vi "InTake Finish.vi"   [LabVIEW 2013]
types:
  T1 = typedef "WPI_MotorControlDeviceRef.ctl" = cluster{"DeviceStatus":errorcluster, "Type":enum16{"PWM", "CAN"}, "PWM":cluster{"Digital Module":T2, "PWM Channel":T3, "DeadBand":T4}, "CAN":cluster{"Device Number":u8, "Control Mode":T5, "Semaphore":T6, "Max Vout":dbl}, "Invert":bool, "TransformRef":T7, "InvTransformRef":T7}
  T2 = typedef "FPGA_TypedefDigitalModule.ctl" = enum16{"Digital Module 1", "Digital Module 2"}
  T3 = typedef "FPGA_DIOPWMChannel.ctl" = enum8{"PWM 1", "PWM 2", "PWM 3", "PWM 4", "PWM 5", "PWM 6", "PWM 7", "PWM 8", "PWM 9", "PWM 10", "Invalid"}
  T4 = typedef "WPI_PWMDeadband.ctl" = cluster{"Name":string, "maxPositivePwm":i32, "minPositivePwm":i32, "centerPwm":i32, "maxNegativePwm":i32, "minNegativePwm":i32, "angularRange":u16}
  T5 = typedef "WPI_CANJaguar_ControlMode.ctl" = enum8{"Percent VBus", "Current", "Speed", "Position", "Voltage"}
  T6 = typedef "Semaphore RefNum" = refnum<k1>
  T7 = typedef "WPI_PWMTransform_ConPane.ctl" = refnum<vi>
  T8 = typedef "WPI_DigitalInputDevRef.ctl" = cluster{"DevStatus":errorcluster, "DIO Channel":T9, "Digital Module":T2}
  T9 = typedef "FPGA_DIOChannel.ctl" = enum8{"DIO 1", "DIO 2", "DIO 3", "DIO 4", "DIO 5", "DIO 6", "DIO 7", "DIO 8", "DIO 9", "DIO 10", "DIO 11", "DIO 12", "DIO 13", "DIO 14", "Invalid"}
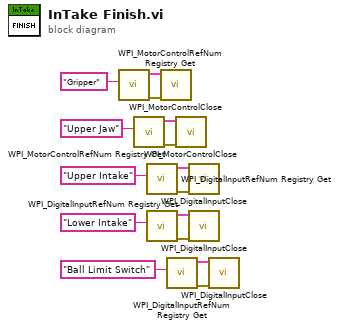
[diagram p0: block diagram]
diagram:
  n1 = call <vilib>:"WPI_MotorControlRefNum Registry Get.vi"("refnum name"="Gripper") -> ("error out"=w10:errorcluster, "MotorControlDevRef"=w9:T1)  [unwired: 9 in]
  n2 = call <vilib>:"WPI_MotorControlRefNum Registry Get.vi"("refnum name"="Upper Jaw") -> ("error out"=w8:errorcluster, "MotorControlDevRef"=w7:T1)  [unwired: 9 in]
  n3 = call <vilib>:"WPI_DigitalInputRefNum Registry Get.vi"("refnum name"="Upper Intake") -> ("error out"=w6:errorcluster, "DigitalInputDevRef"=w5:T8)  [unwired: 9 in]
  n4 = call <vilib>:"WPI_DigitalInputRefNum Registry Get.vi"("refnum name"="Lower Intake") -> ("error out"=w4:errorcluster, "DigitalInputDevRef"=w3:T8)  [unwired: 9 in]
  n5 = call <vilib>:"WPI_MotorControlClose.vi"("error in (no error)"=w10, "MotorControlDevRef"=w9) -> ()  [unwired: 9 in, 1 out]
  n6 = call <vilib>:"WPI_DigitalInputRefNum Registry Get.vi"("refnum name"="Ball Limit Switch") -> ("error out"=w1:errorcluster, "DigitalInputDevRef"=w2:T8)  [unwired: 9 in]
  n7 = call <vilib>:"WPI_MotorControlClose.vi"("error in (no error)"=w8, "MotorControlDevRef"=w7) -> ()  [unwired: 9 in, 1 out]
  n8 = call <vilib>:"WPI_DigitalInputClose.vi"("error in (no error)"=w6, "DigitalInputDevRef"=w5) -> ()  [unwired: 9 in, 1 out]
  n9 = call <vilib>:"WPI_DigitalInputClose.vi"("error in (no error)"=w4, "DigitalInputDevRef"=w3) -> ()  [unwired: 9 in, 1 out]
  n10 = call <vilib>:"WPI_DigitalInputClose.vi"("error in (no error)"=w1, "DigitalInputDevRef"=w2) -> ()  [unwired: 9 in, 1 out]
